vi "Create Top Level.vi"(9 "Alias":string, 10 "Actor":refnum<class "Actor.lvclass">) -> ()   [LabVIEW 2021, in "jettl.lvlib" / "Self Actor.lvclass"]
uses:
  Self Actor.lvclass
  Actor/Actor.lvclass
  Self Actor.lvclass/Self Actor.ctl
  jettl.lvlib
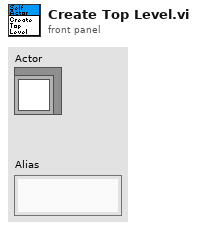
[diagram p1: front panel]
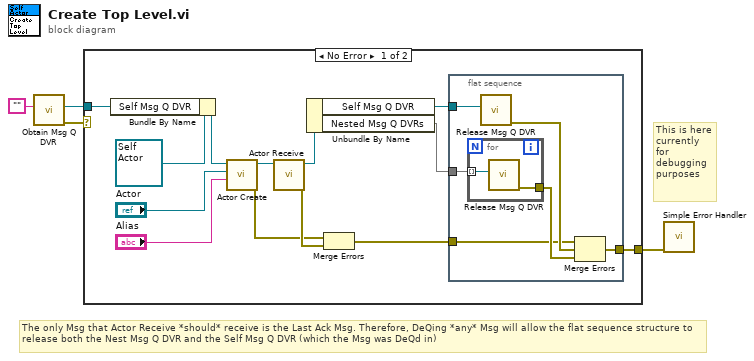
[diagram p0: block diagram]
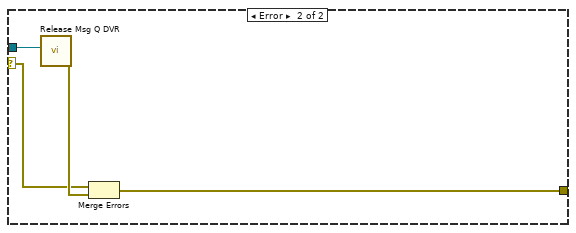
[diagram p2: hidden frame]
diagram:
  # "This is here currently for debugging purposes"
  # "The only Msg that Actor Receive *should* receive is the Last Ack Msg. Therefore, DeQing *any* Msg will allow the flat sequence structure to release both the Nest Msg Q DVR and the Self Msg Q DVR (which the Msg was DeQd in)"
  n1 = call "Obtain Msg Q DVR.vi"("Msg Q DVR Alias"="") -> ("error out"=w1:errorcluster, "Msg Q DVR"=w4:refnum<data-value>)  [unwired: 9 in]
  n2 = case shown="No Error" w1 {
    selector: w1 -> [_ w26]
    tunnel: w4 -> [w16 w29]
    tunnel: [w15 w28] -> w3
    frame No Error {
      n3 = Bundle By Name(cluster=refnum<class "Self Actor.lvclass"> refnum ("Self Actor in"), "Self Msg Q DVR"=w16) -> (w12:refnum<class "Self Actor.lvclass">)
      n4 = call-dynamic "Actor Create.vi"("Nested Alias"="Alias", "Nested Actor"="Actor", "Self Actor in"=w12) -> ("error out"=w7:errorcluster, "Self Actor out"=w6:refnum<class "Self Actor.lvclass">)  [unwired: 7 in]
      n5 = call-dynamic "Actor Receive.vi"("Self Actor in"=w6) -> ("error out"=w8:errorcluster, "Self Actor out"=w5:refnum<class "Self Actor.lvclass">)  [unwired: 8 in, 1 out]
      n6 = Unbundle By Name(w5) -> ("Self Msg Q DVR"=w17:refnum<data-value>, "Nested Msg Q DVRs"=w14:set{refnum<data-value>})
      n7 = Merge Errors(w7, w8) -> (w13:errorcluster)
      n8 = flat-sequence {
        tunnel: w17 -> [w23]
        tunnel: [w22] -> w15
        tunnel: w14 -> [w21]
        tunnel: w13 -> [w18]
        frame #0 {
          n9 = for {
            tunnel: w21 -> [w25] mode=indexing
            tunnel: [w24] -> w20
            n10 = call "Release Msg Q DVR.vi"("Msg Q DVR"=w25) -> ("error out"=w24:errorcluster)  [unwired: 10 in]
          }
          n11 = call "Release Msg Q DVR.vi"("Msg Q DVR"=w23) -> ("error out"=w19:errorcluster)  [unwired: 10 in]
          n12 = Merge Errors(w18, w19, w20) -> (w22:errorcluster)
        }
      }
    }
    frame Error {
      n13 = call "Release Msg Q DVR.vi"("Msg Q DVR"=w29) -> ("error out"=w27:errorcluster)  [unwired: 10 in]
      n14 = Merge Errors(w26, w27) -> (w28:errorcluster)
    }
  }
  n15 = call <vilib>:"Simple Error Handler.vi"("error in (no error)"=w3) -> ()  [unwired: 4 in, 5 out]
